vi "Out_S6F19.vi"(8 "error in (no error)":errorcluster, 10 "RPTID":u32, 11 "S6 Message Class in":refnum<class "S6 Message Class.lvclass">) -> (0 "error out":errorcluster, 3 "S6 Message Class out":refnum<class "S6 Message Class.lvclass">)   [LabVIEW 2020, in "SECS Communication.lvlib" / "S6 Message Class.lvclass"]
uses:
  S6 Message Class.lvclass
  D:/Dropbox/SECS/SECS_GEM v1.0.6/Com/SECS Communication/SECS-II Class/SECS-II Class.lvclass
  SECS-II Class/Data Message_U4.vi
  SECS-II Class/SECS-II Class.lvclass
  D:/Dropbox/SECS/SECS_GEM v1.0.6/Com/SECS Communication/S6 Message Class/S6 Message Class.lvclass
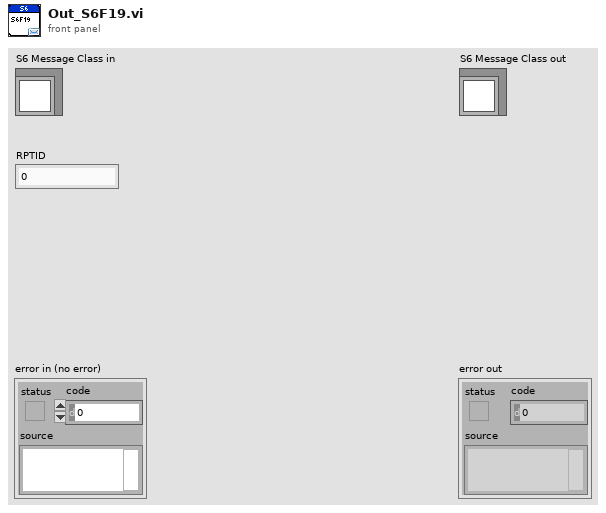
[diagram p1: front panel]
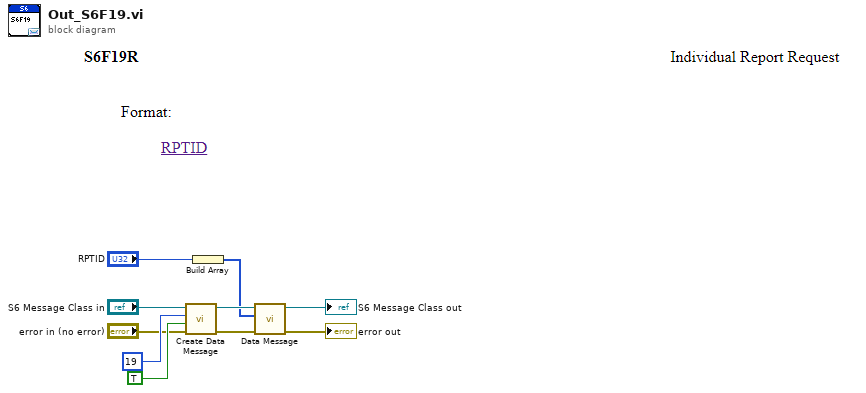
[diagram p0: block diagram]
diagram:
  n1 = call "Create Data Message.vi"("error in (no error)"="error in (no error)", "W-Bit"=TRUE, "Function"=u8 19, "SECS-II Class in"="S6 Message Class in") -> ("error out"=w7:errorcluster, "SECS-II Class out"=w8:refnum<class "S6 Message Class.lvclass">)  [unwired: 6 in]
  n2 = Build Array("RPTID") -> (w3:u32[])
  n3 = call-poly "Data Message.vi"("error in"=w7, "Data"=w3, "SECS-II Class in"=w8) -> ("error out"=→"error out":errorcluster, "SECS-II Class out"=→"S6 Message Class out":refnum<class "S6 Message Class.lvclass">)  [unwired: 7 in]
